vi "Get All Charact Results.vi"(11 "error in":errorcluster) -> (4 "All Cal Results":variant[](array[variant]), 15 "error out":errorcluster)   [LabVIEW 2023, in "RFFixtureCharact.Public.lvlib"]
uses:
  RFFixtureCharact.Public.lvlib
  Type Definitions/Collection Operation.ctl
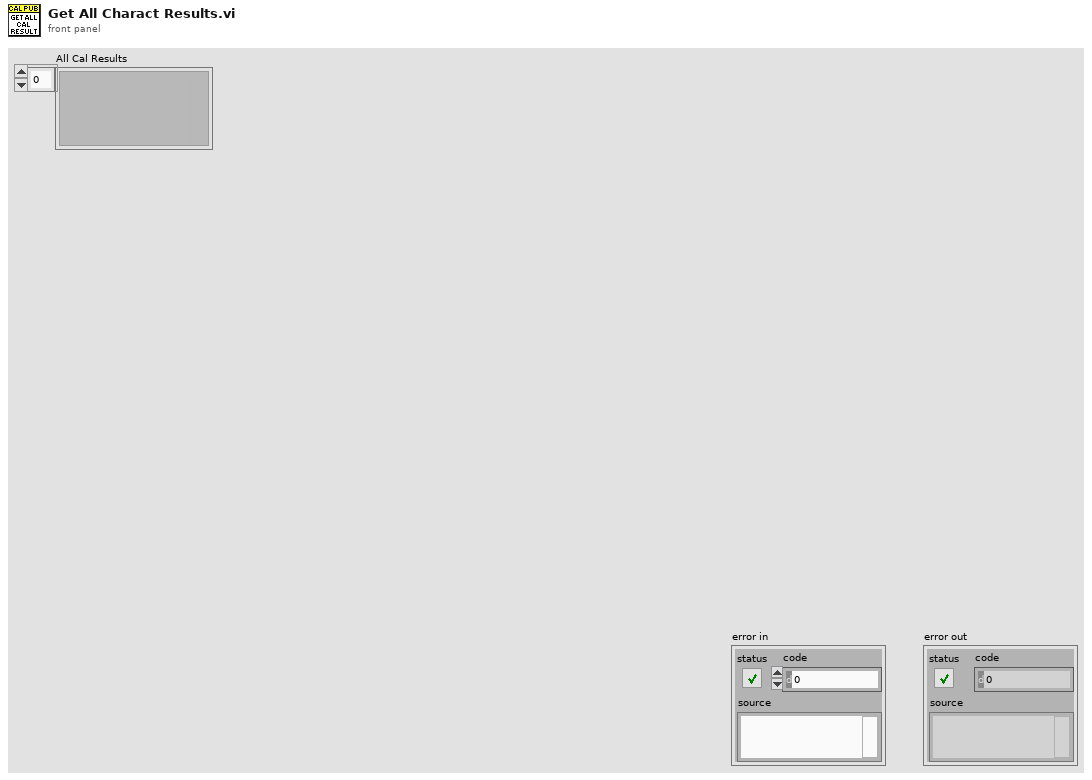
[diagram p1: front panel]
types:
  T1 = typedef "RFFixtureCharact.Public.lvlib/Collection Operation.ctl" = enum16{"Append", "Get", "Get All", "Clear"}
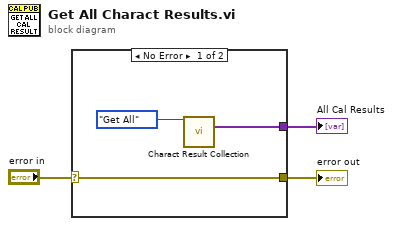
[diagram p0: block diagram]
diagram:
  n1 = case shown="No Error" "error in" {
    selector: "error in" -> [w4 w7]
    tunnel: [w5 _] -> w3
    tunnel: [w4 w7] -> w1
    frame No Error {
      n2 = call "Charact Result Collection.vi"("Operation"=Collection_Operation."Get All") -> ("All path cal results"=w5:variant[])  [unwired: 13 in, 1 out]
    }
    frame Error {
    }
  }
  "All Cal Results" <- w3
  "error out" <- w1
